vi "srednia.vi"(11 "Array":dbl[](array[numeric])) -> (1 "RMS":dbl, 2 "Sredniokwadratowa":dbl, 3 "Srednia":dbl)   [LabVIEW 2019]
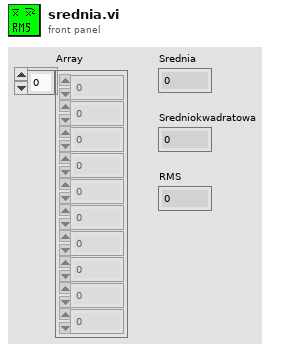
[diagram p1: front panel]
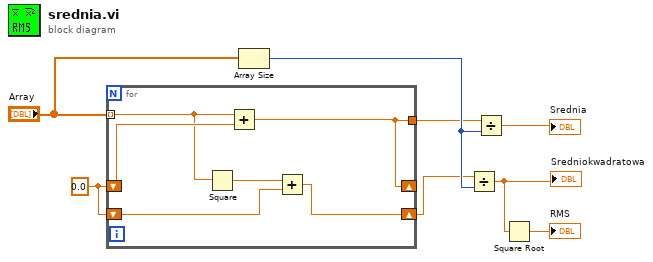
[diagram p0: block diagram]
diagram:
  w3 = 0.0
  n1 = for {
    tunnel: "Array" -> [w9] mode=indexing
    shift-right: [w13] -> _
    shift-left: w3 -> [w14]
    tunnel: [w13] -> w1
    shift-right: [w12] -> w4
    shift-left: w3 -> [w11]
    n2 = Square(x=w9) -> (x^2=w10:dbl)
    n3 = Add(x=w9, y=w14) -> (x+y=w13:dbl)
    n4 = Add(x=w10, y=w11) -> (x+y=w12:dbl)
  }
  n5 = Array Size(array="Array") -> (size(s)=w5:i32)
  n6 = Divide(x=w4, y=w5) -> (x/y=w6:dbl)
  "Sredniokwadratowa" <- w6
  n7 = Divide(x=w1, y=w5) -> (x/y=→"Srednia":dbl)
  n8 = Square Root(x=w6) -> (sqrt(x)=→"RMS":dbl)
